vi "QControl Creation Wizard.vi"(10 "ProjectItemRefnum":refnum<vi>, 11 "App Refnum":refnum<vi>) -> ()   [LabVIEW 2015, in "QControl Creation Wizard.lvclass"]
doc: "<b> </b> <b> </b>\n©2016 Q Software Innovations, LLC (QSI)\nwritten by Quentin Alldredge\nproduced in LabVIEW 2015\n\nsupport@qsoftwareinnovations.com\nwww.qsoftwareinnovations.com\n\nAll rights reserved.\n\nRedistribution and use in source and binary forms, with or without modification, are permitted provided that the following conditions are met:\n\n * Redistributions of source code must retain the above copyright notice, this list of conditions and the following disclaimer.\n * Redistributions in binary form must reproduce the above copyright notice, this list of conditions and the following disclaimer in the documentation and/or other materials provided with the distribution.\n * Neither the name of Q Software Innovations, LLC. nor the names of its contributors may be used to endorse or promote products derived from this software without specific prior written permission.\n\nTHIS SOFTWARE IS PROVIDED BY THE COPYRIGHT HOLDERS AND CONTRIBUTORS \"AS IS\" AND ANY EXPRESS OR IMPLIED WARRANTIES, INCLUDING, BUT NOT LIMITED TO, THE IMPLIED WARRANTIES OF MERCHANTABILITY AND FITNESS FOR A PARTICULAR PURPOSE ARE DISCLAIMED. IN NO EVENT SHALL THE COPYRIGHT OWNER OR CONTRIBUTORS BE LIABLE FOR ANY DIRECT, INDIRECT, INCIDENTAL, SPECIAL, EXEMPLARY, OR CONSEQUENTIAL DAMAGES (INCLUDING, BUT NOT LIMITED TO, PROCUREMENT OF SUBSTITUTE GOODS OR SERVICES; LOSS OF USE, DATA, OR PROFITS; OR BUSINESS INTERRUPTION) HOWEVER CAUSED AND ON ANY THEORY OF LIABILITY, WHETHER IN CONTRACT, STRICT LIABILITY, OR TORT (INCLUDING NEGLIGENCE OR OTHERWISE) ARISING IN ANY WAY OUT OF THE USE OF THIS SOFTWARE, EVEN IF ADVISED OF THE POSSIBILITY OF SUCH DAMAGE."
uses:
  QControl Creation Wizard.lvclass
  New QControl Info/New QControl Info.lvclass/New QControl Info.ctl
  QControl Creation Wizard.lvclass/QControl Creation Wizard.ctl
  <vilib>/Utility/error.llb/DialogType.ctl
  New QControl Info/Write App Refnum.vi
  New QControl Info/Read StatusUpdate.vi
  New QControl Info/Read CreatorComplete.vi
  QControl Classes/StatusHistory/Add Item.vi
  <vilib>/Utility/error.llb/Error Cluster From Error Code.vi
  <vilib>/ErrorRing/Error Ring.xnode
  QControl Classes/Steps/Steps.lvclass
  QControl Classes/TreeSelectionSingle/TreeSelectionSingle.lvclass
  QControl Classes/StatusHistory/StatusHistory.lvclass
  New QControl Info/New QControl Info.lvclass
panel:
  out "Help Message":string="For more help click the \nHelp Menu->QSI-> QControl Toolkit Help...\nor find examples in the NI Example Finder."
  in  "Explore":bool
  in  "Back":bool
  in  "Steps":T1(tab)
  in  "ParentPath":path
  in  "QControl Class Hierarchy":string(tree)
  in  "Inheritance":enum32{"Tree", "Path"}(radio)
  in  "Class Name":string caption="QControl Name *"
  in  "Localized Name":string caption="Localized Name *"
  in  "Description":string
  out "New Class Data Icon":picture
  in  "Banner Text":string caption="Banner Text *"
  out "New Class Banner":picture
  out "Final Path":path
  in  "Save Location":path
  out "Status":string
  in  "Next":bool
  # "QControl Creation Wizard"
  # "©2016,2021 Q Software Innovations, LLC\nsupport@qsoftwareinnovations.com\n\nQControl Creation Wizard is distributed\nfree as part of the QControl Toolkit"
  # "Click Next to Begin"
  # "Choose the class to inherit from:\n      Select from the tree OR browse to the path of the class to inherit from."
  # "* Required Field"
  # "(Recommend 6 Characters or Fewer)"
  # "Icon Preview"
  # "* Required Field"
  # "Choose where to save your new QControl."
  # "A new folder with the QControl's name will be appended to this path automatically."
  # "The final path will be:"
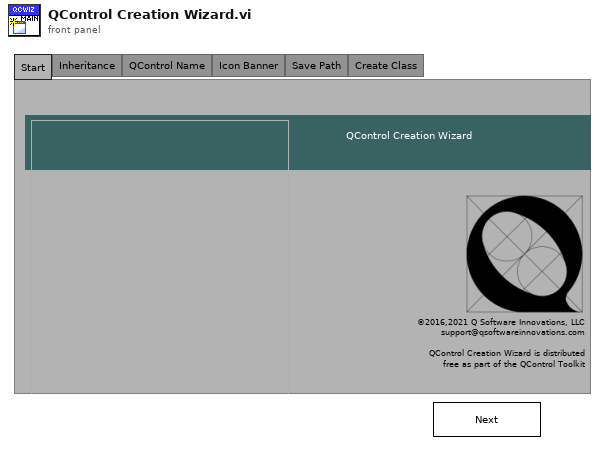
[diagram p1: front panel]
types:
  T1 = enum32{"Start", "Inheritance", "QControl Name", "Icon Banner", "Save Path", "Create Class"}
  T2 = typedef "LVPoint32TypeDef.ctl" = cluster{"Horizontal":i32, "Vertical":i32}
  T3 = typedef "DialogType.ctl" = u16
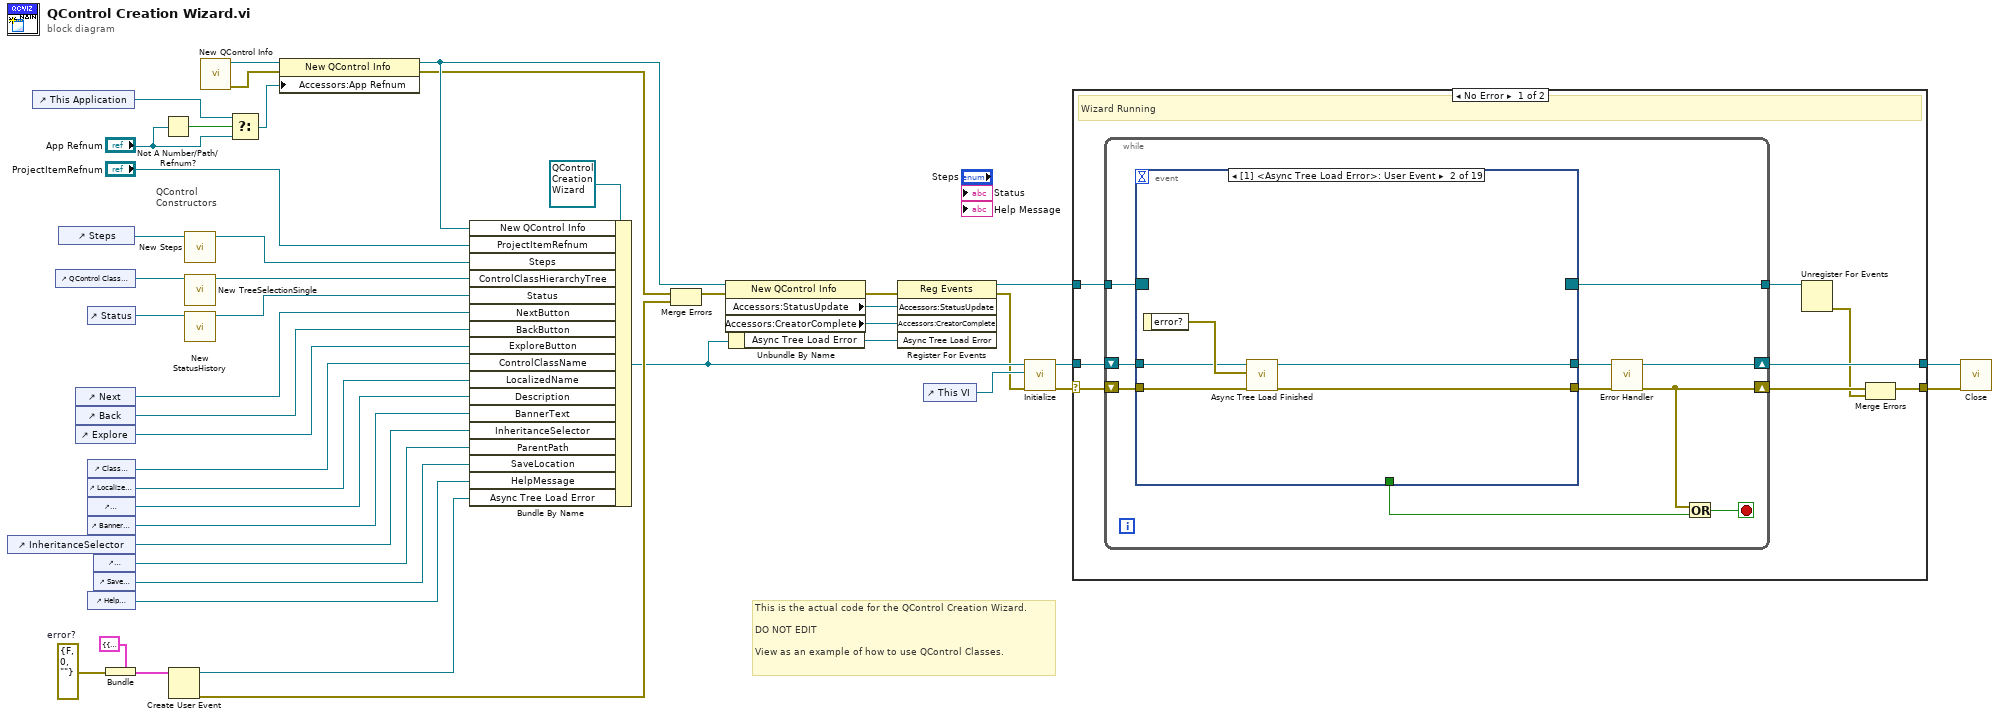
[diagram p0: block diagram]
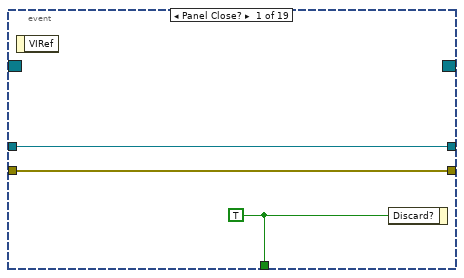
[diagram p2: hidden frame]
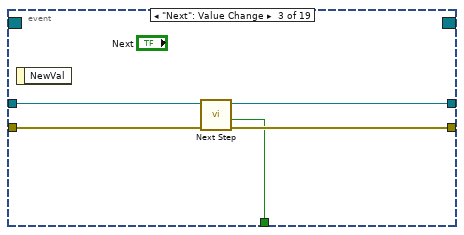
[diagram p3: hidden frame]
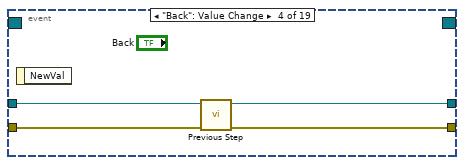
[diagram p4: hidden frame]
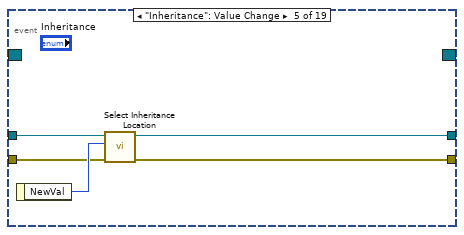
[diagram p5: hidden frame]
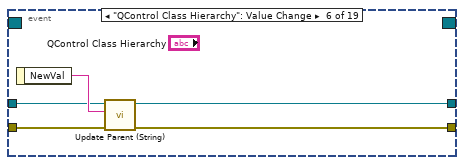
[diagram p6: hidden frame]
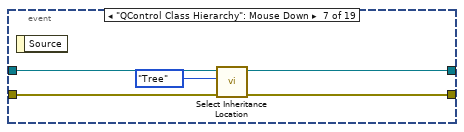
[diagram p7: hidden frame]
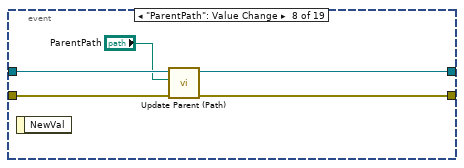
[diagram p8: hidden frame]
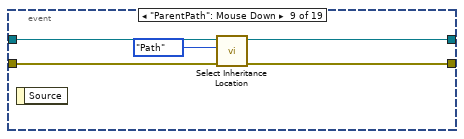
[diagram p9: hidden frame]
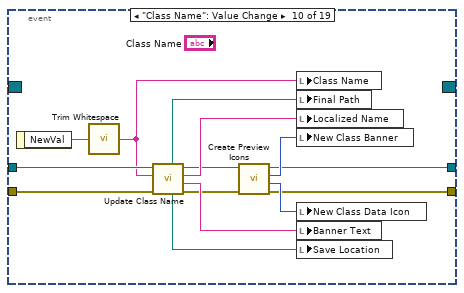
[diagram p10: hidden frame]
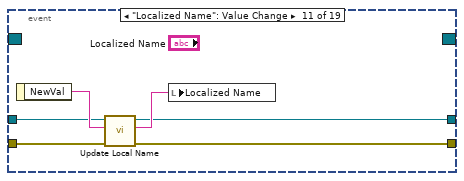
[diagram p11: hidden frame]
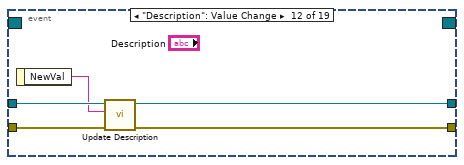
[diagram p12: hidden frame]
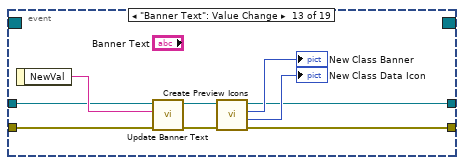
[diagram p13: hidden frame]
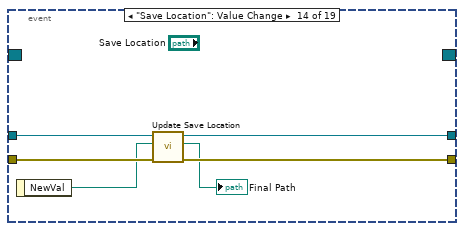
[diagram p14: hidden frame]
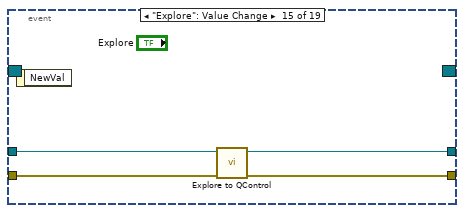
[diagram p15: hidden frame]
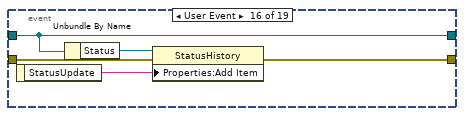
[diagram p16: hidden frame]
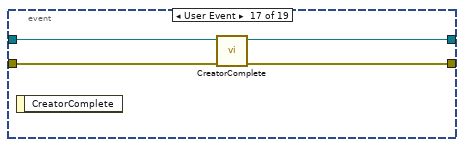
[diagram p17: hidden frame]
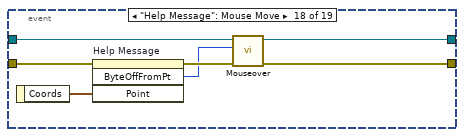
[diagram p18: hidden frame]
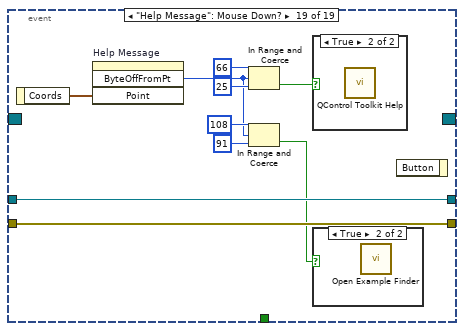
[diagram p19: hidden frame]
diagram:
  w9 = errorcluster {"status"=FALSE, "code"=0, "source"=""}  # error?
  # "This is the actual code for the QControl Creation Wizard.\n\nDO NOT EDIT\n\nView as an example of how to use QControl Classes."
  # "QControl\nConstructors"
  n1 = control-ref of="InheritanceSelector"() -> (w38:refnum<vi>)
  n2 = control-ref of="This Application"() -> (w31:refnum<vi>)
  n3 = control-ref of="QControl Class Hierarchy"() -> (w25:refnum<vi>)
  n4 = control-ref of="Steps"() -> (w26:refnum<vi>)
  n5 = control-ref of="Next"() -> (w43:refnum<vi>)
  n6 = control-ref of="Back"() -> (w42:refnum<vi>)
  n7 = control-ref of="Explore"() -> (w35:refnum<vi>)
  n8 = control-ref of="Status"() -> (w23:refnum<vi>)
  n9 = control-ref of="Class Name"() -> (w41:refnum<vi>)
  n10 = control-ref of="Localized Name"() -> (w36:refnum<vi>)
  n11 = control-ref of="Description"() -> (w34:refnum<vi>)
  n12 = control-ref of="Banner Text"() -> (w40:refnum<vi>)
  n13 = control-ref of="Help Message"() -> (w21:refnum<vi>)
  n14 = control-ref of="ParentPath"() -> (w39:refnum<vi>)
  n15 = control-ref of="Save Location"() -> (w37:refnum<vi>)
  n16 = Bundle(cluster=cluster{"error?":errorcluster} {"error?"={"status"=FALSE, "code"=0, "source"=""}}, "error?"=w9) -> (w10:cluster{"error?":errorcluster})
  n17 = Not A Number/Path/Refnum?(number/path/refnum="App Refnum") -> (NaN/Path/Refnum?=w32:bool)
  n18 = Create User Event(user event datatype=w10) -> (user event=w8:refnum<user-event>, error out=w5:errorcluster)  [unwired: 1 in]
  n19 = call "New Steps.vi"("Reference"=w26) -> ("Steps out"=w27:refnum<class "Steps.lvclass">)  [unwired: 9 in, 1 out]
  n20 = call "New TreeSelectionSingle.vi"("Reference"=w25) -> ("TreeSelectionSingle out"=w24:refnum<class "TreeSelectionSingle.lvclass">)  [unwired: 9 in, 1 out]
  n21 = call "New StatusHistory.vi"("Reference"=w23) -> ("StatusHistory out"=w22:refnum<class "StatusHistory.lvclass">)  [unwired: 9 in, 1 out]
  n22 = call "New QControl Info.vi"() -> ("error out"=w13:errorcluster, "New QControl Info"=w20:refnum<data-value>)  [unwired: 8 in, 2 out]
  n23 = Select(t=w31, s=w32, f="App Refnum") -> (s? t:f=w19:refnum<vi>)
  n24 = property class="New QControl Info"(reference=w20, error in=w13, "Accessors:App Refnum"=w19) -> (reference out=w18:refnum<data-value>, error out=w7:errorcluster)
  n25 = Bundle By Name(cluster=refnum<class "QControl Creation Wizard.lvclass"> refnum ("ControlClassWizard"), "New QControl Info"=w18, "ProjectItemRefnum"="ProjectItemRefnum", "Steps"=w27, "ControlClassHierarchyTree"=w24, "Status"=w22, "NextButton"=w43, "BackButton"=w42, "ExploreButton"=w35, "ControlClassName"=w41, "LocalizedName"=w36, "Description"=w34, "BannerText"=w40, "InheritanceSelector"=w38, "ParentPath"=w39, "SaveLocation"=w37, "HelpMessage"=w21, "Async Tree Load Error"=w8) -> (w4:refnum<class "QControl Creation Wizard.lvclass">)
  n26 = Merge Errors(w7, w5) -> (w6:errorcluster)
  n27 = property class="New QControl Info"(reference=w18, error in=w6) -> (error out=w15:errorcluster, "Accessors:StatusUpdate"=w17:refnum<user-event>, "Accessors:CreatorComplete"=w16:refnum<user-event>)  [unwired: 1 out]
  n28 = Unbundle By Name(w4) -> ("Async Tree Load Error"=w12:refnum<user-event>)
  n29 = register-events(error in=w15, w17, w16, w12) -> (reference out=w28:refnum<event-registration>, error out=w2:errorcluster)  [unwired: 1 in]
  n30 = control-ref of="This VI"() -> (w33:refnum<vi>)
  n31 = call-dynamic "Initialize.vi"("error in (no error)"=w2, "VI Refnum"=w33, "ControlClassWizard in"=w4) -> ("error out"=w1:errorcluster, "ControlClassWizard out"=w3:refnum<class "QControl Creation Wizard.lvclass">)  [unwired: 7 in]
  n32 = case shown="No Error" w1 {
    selector: w1 -> [w49 w182]
    tunnel: [w53 w178] -> w45
    tunnel: [w47 w177] -> w44
    tunnel: w28 -> [w51 _]
    tunnel: w3 -> [w50 w181]
    frame No Error {
      # "Wizard Running"
      n33 = while {
        shift-right: [w57] -> w53
        shift-left: w50 -> [w63]
        shift-right: [w55] -> w52
        shift-left: w49 -> [w62]
        tunnel: w51 -> [w59]
        tunnel: [w54] -> w48
        stop <- w60 stop-if-true
        n34 = event shown="[1] <Async Tree Load Error>: User Event" {
          selector: w59 -> [_ _ _ _ _ _ _ _ _ _ _ _ _ _ _ _ _ _ _]
          dyn-events: [_ _ _ _ _ _ _ _ _ _ _ _ _ _ _ _ _ _ _] -> w54
          timeout: _ -> [_ _ _ _ _ _ _ _ _ _ _ _ _ _ _ _ _ _ _]
          tunnel: w63 -> [w66 w67 w76 w80 w84 w89 w95 w100 w105 w117 w124 w130 w132 w145 w147 w151 w158 w165 w175]
          tunnel: w62 -> [w65 w71 w75 w79 w82 w88 w93 w98 w103 w119 w123 w129 w139 w144 w149 w152 w156 w162 w174]
          tunnel: [w66 w68 w74 w78 w83 w87 w94 w97 w104 w111 w121 w127 w133 w143 w146 w151 w157 w164 w175] -> w58
          tunnel: [w65 w69 w73 w77 w81 w86 w92 w96 w102 w109 w120 w126 w131 w142 w148 w150 w155 w159 w174] -> w56
          tunnel: [w64 _ w72 _ _ _ _ _ _ _ _ _ _ _ _ _ _ _ _] -> w61
          event Panel Close? {
            w64 = TRUE ("Discard?")
            n35 = event-data() -> ()  [unwired: 1 in, 1 out]
            n36 = event-data("Discard?"=w64) -> ()  [unwired: 1 in, 1 out]
          }
          event User Event {
            n37 = event-data() -> ("error?"=w70:errorcluster)  [unwired: 1 in]
            n38 = call "Async Tree Load Finished.vi"("error in (no error)"=w71, "error?"=w70, "QControlWizard in"=w67) -> ("error out"=w69:errorcluster, "QControlWizard out"=w68:refnum<class "QControl Creation Wizard.lvclass">)  [unwired: 7 in]
          }
          event "Next": Value Change {
            n39 = event-data() -> ()  [unwired: 1 in, 1 out]
            n40 = call "Next Step.vi"("error in (no error)"=w75, "ControlClassWizard in"=w76) -> ("error out"=w73:errorcluster, "Finish Button?"=w72:bool, "ControlClassWizard out"=w74:refnum<class "QControl Creation Wizard.lvclass">)  [unwired: 6 in, 1 out]
          }
          event "Back": Value Change {
            n41 = event-data() -> ()  [unwired: 1 in, 1 out]
            n42 = call "Previous Step.vi"("error in (no error)"=w79, "ControlClassWizard in"=w80) -> ("error out"=w77:errorcluster, "ControlClassWizard out"=w78:refnum<class "QControl Creation Wizard.lvclass">)  [unwired: 8 in]
          }
          event "Inheritance": Value Change {
            n43 = event-data() -> ("NewVal"=w85:enum32{"Tree", "Path"})  [unwired: 1 in]
            n44 = call "Select Inheritance Location.vi"("error in (no error)"=w82, "NewVal"=w85, "QControlWizard in"=w84) -> ("error out"=w81:errorcluster, "QControlWizard (dup)"=w83:refnum<class "QControl Creation Wizard.lvclass">)  [unwired: 7 in]
          }
          event "QControl Class Hierarchy": Value Change {
            n45 = event-data() -> ("NewVal"=w90:string)  [unwired: 1 in]
            n46 = call "Update Parent (String).vi"("error in (no error)"=w88, "Parent Name"=w90, "ControlClassWizard in"=w89) -> ("error out"=w86:errorcluster, "ControlClassWizard (dup)"=w87:refnum<class "QControl Creation Wizard.lvclass">)  [unwired: 7 in]
          }
          event "QControl Class Hierarchy": Mouse Down {
            n47 = event-data() -> ()  [unwired: 1 in, 1 out]
            n48 = call "Select Inheritance Location.vi"("error in (no error)"=w93, "NewVal"=enum32{"Tree", "Path"}."Tree", "QControlWizard in"=w95) -> ("error out"=w92:errorcluster, "QControlWizard (dup)"=w94:refnum<class "QControl Creation Wizard.lvclass">)  [unwired: 7 in]
          }
          event "ParentPath": Value Change {
            n49 = event-data() -> ()  [unwired: 1 in, 1 out]
            n50 = call "Update Parent (Path).vi"("error in (no error)"=w98, "Parent Path"="ParentPath", "ControlClassWizard in"=w100) -> ("error out"=w96:errorcluster, "ControlClassWizard (dup)"=w97:refnum<class "QControl Creation Wizard.lvclass">)  [unwired: 7 in]
          }
          event "ParentPath": Mouse Down {
            n51 = event-data() -> ()  [unwired: 1 in, 1 out]
            n52 = call "Select Inheritance Location.vi"("error in (no error)"=w103, "NewVal"=enum32{"Tree", "Path"}."Path", "QControlWizard in"=w105) -> ("error out"=w102:errorcluster, "QControlWizard (dup)"=w104:refnum<class "QControl Creation Wizard.lvclass">)  [unwired: 7 in]
          }
          event "Class Name": Value Change {
            n53 = event-data() -> ("NewVal"=w108:string)  [unwired: 1 in]
            n54 = call <vilib>:"Trim Whitespace.vi"("string"=w108) -> ("trimmed string"=w107:string)  [unwired: 1 in]
            n55 = call "Update Class Name.vi"("error in (no error)"=w119, "Class Name"=w107, "ControlClassWizard in"=w117) -> ("error out"=w113:errorcluster, "Banner Text"=w115:string, "Localized Name"=w118:string, "ControlClassWizard out"=w114:refnum<class "QControl Creation Wizard.lvclass">, "Save Location"=w116:path, "Final Path"=w106:path)  [unwired: 3 in]
            n56 = call "Create Preview Icons.vi"("error in (no error)"=w113, "ControlClassWizard in"=w114) -> ("error out"=w109:errorcluster, "Class Data Icon"=w110:picture, "Class Banner Icon"=w112:picture, "ControlClassWizard (dup)"=w111:refnum<class "QControl Creation Wizard.lvclass">)  [unwired: 6 in]
            n57 = local write "Class Name"(w107) -> ()
            n58 = local write "Final Path"(w106) -> ()
            n59 = local write "Localized Name"(w118) -> ()
            n60 = local write "New Class Banner"(w112) -> ()
            n61 = local write "New Class Data Icon"(w110) -> ()
            n62 = local write "Banner Text"(w115) -> ()
            n63 = local write "Save Location"(w116) -> ()
          }
          event "Localized Name": Value Change {
            n64 = event-data() -> ("NewVal"=w125:string)  [unwired: 1 in]
            n65 = call "Update Local Name.vi"("error in (no error)"=w123, "Localized Name"=w125, "ControlClassWizard in"=w124) -> ("error out"=w120:errorcluster, "Localized Name"=w122:string, "ControlClassWizard (dup)"=w121:refnum<class "QControl Creation Wizard.lvclass">)  [unwired: 6 in]
            n66 = local write "Localized Name"(w122) -> ()
          }
          event "Description": Value Change {
            n67 = event-data() -> ("NewVal"=w128:string)  [unwired: 1 in]
            n68 = call "Update Description.vi"("error in (no error)"=w129, "Description"=w128, "ControlClassWizard in"=w130) -> ("error out"=w126:errorcluster, "ControlClassWizard (dup)"=w127:refnum<class "QControl Creation Wizard.lvclass">)  [unwired: 7 in]
          }
          event "Banner Text": Value Change {
            n69 = event-data() -> ("NewVal"=w134:string)  [unwired: 1 in]
            n70 = call "Update Banner Text.vi"("error in (no error)"=w139, "Banner Text"=w134, "ControlClassWizard in"=w132) -> ("error out"=w138:errorcluster, "ControlClassWizard (dup)"=w137:refnum<class "QControl Creation Wizard.lvclass">)  [unwired: 7 in]
            n71 = call "Create Preview Icons.vi"("error in (no error)"=w138, "ControlClassWizard in"=w137) -> ("error out"=w131:errorcluster, "Class Data Icon"=→"New Class Data Icon":picture, "Class Banner Icon"=→"New Class Banner":picture, "ControlClassWizard (dup)"=w133:refnum<class "QControl Creation Wizard.lvclass">)  [unwired: 6 in]
          }
          event "Save Location": Value Change {
            n72 = event-data() -> ("NewVal"=w141:path)  [unwired: 1 in]
            n73 = call "Update Save Location.vi"("error in (no error)"=w144, "Path"=w141, "ControlClassWizard in"=w145) -> ("error out"=w142:errorcluster, "Final Path out"=→"Final Path":path, "ControlClassWizard out"=w143:refnum<class "QControl Creation Wizard.lvclass">)  [unwired: 6 in]
          }
          event "Explore": Value Change {
            n74 = event-data() -> ()  [unwired: 1 in, 1 out]
            n75 = call "Explore to QControl.vi"("error in (no error)"=w149, "ControlClassWizard in"=w147) -> ("error out"=w148:errorcluster, "ControlClassWizard (dup)"=w146:refnum<class "QControl Creation Wizard.lvclass">)  [unwired: 8 in]
          }
          event User Event {
            n76 = event-data() -> ("StatusUpdate"=w154:string)  [unwired: 1 in]
            n77 = Unbundle By Name(w151) -> ("Status"=w153:refnum<class "StatusHistory.lvclass">)
            n78 = property class="StatusHistory"(reference=w153, error in=w152, "Properties:Add Item"=w154) -> (error out=w150:errorcluster)  [unwired: 1 out]
          }
          event User Event {
            n79 = event-data() -> ()  [unwired: 1 in, 1 out]
            n80 = call "CreatorComplete.vi"("error in (no error)"=w156, "QControlWizard in"=w158) -> ("error out"=w155:errorcluster, "QControlWizard (dup)"=w157:refnum<class "QControl Creation Wizard.lvclass">)  [unwired: 8 in]
          }
          event "Help Message": Mouse Move {
            n81 = event-data() -> ("Coords"=w163:T2)  [unwired: 1 in]
            n82 = invoke on="Help Message" class="Str" method="ByteOffFromPt"(error in=w162, "Point"=w163) -> (error out=w161:errorcluster, "ByteOffFromPt"=w160:i32)  [unwired: 2 in, 2 out]
            n83 = call "Mouseover.vi"("error in (no error)"=w161, "Byte Offset from Point"=w160, "QControlWizard in"=w165) -> ("error out"=w159:errorcluster, "QControlWizard out"=w164:refnum<class "QControl Creation Wizard.lvclass">)  [unwired: 7 in]
          }
          event "Help Message": Mouse Down? {
            n84 = event-data() -> ("Coords"=w173:T2)  [unwired: 1 in]
            n85 = invoke on="Help Message" class="Str" method="ByteOffFromPt"("Point"=w173) -> ("ByteOffFromPt"=w167:i32)  [unwired: 3 in, 3 out]
            n86 = In Range and Coerce(upper limit=66, x=w167, lower limit=25) -> (In Range?=w170:bool)  [unwired: 1 out]
            n87 = In Range and Coerce(upper limit=108, x=w167, lower limit=91) -> (In Range?=w166:bool)  [unwired: 1 out]
            n88 = case shown="True" w170 {
              frame False {
              }
              frame True {
                n89 = call "QControl Toolkit Help.vi"() -> ()  [unwired: 12 in]
              }
            }
            n90 = case shown="True" w166 {
              frame False {
              }
              frame True {
                n91 = call "Open Example Finder.vi"() -> ()  [unwired: 2 in]
              }
            }
            n92 = event-data() -> ()  [unwired: 2 in, 1 out]
          }
        }
        n93 = call "Error Handler.vi"("error in (no error)"=w56, "QControlWizard in"=w58) -> ("error out"=w55:errorcluster, "QControlWizard out"=w57:refnum<class "QControl Creation Wizard.lvclass">)  [unwired: 8 in]
        n94 = Or(x=w55, y=w61) -> (x .or. y?=w60:bool)
      }
      n95 = Unregister For Events(event registration refnum=w48) -> (error out=w46:errorcluster)  [unwired: 1 in]
      n96 = Merge Errors(w52, w46) -> (w47:errorcluster)
    }
    frame Error {
      w176 = T3 0 items=["no dialog", "OK message", "continue or stop message", "OK message + warnings", "continue/stop + warnings"] ("type of dialog (OK msg:1)")
      # "Error Occured on Initialization.  This shouldn't happen.  This is here for development time."
      n97 = call <vilib>:"Simple Error Handler.vi"("type of dialog (OK msg:1)"=w176, "error in (no error)"=w182) -> ("message"=w180:string)  [unwired: 3 in, 4 out]
      n98 = xnode "Error Ring"("parameter 0"=w180) -> ("error out"=w179:errorcluster)
      n99 = call "Error Handler.vi"("error in (no error)"=w179, "QControlWizard in"=w181) -> ("error out"=w177:errorcluster, "QControlWizard out"=w178:refnum<class "QControl Creation Wizard.lvclass">)  [unwired: 8 in]
    }
  }
  n100 = call-dynamic "Close.vi"("error in (no error)"=w44, "ControlClassWizard in"=w45) -> ()  [unwired: 9 in, 1 out]
